vi "XYZArrayInverter.vi"(1 "input array":dbl[](array[numeric]), 2 "invert?":bool, 3 "Number":i32) -> (0 "modified array":dbl[](array[numeric]))   [LabVIEW 2015]
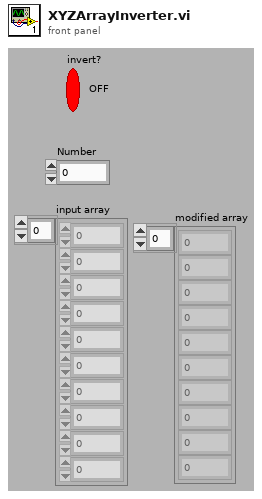
[diagram p1: front panel]
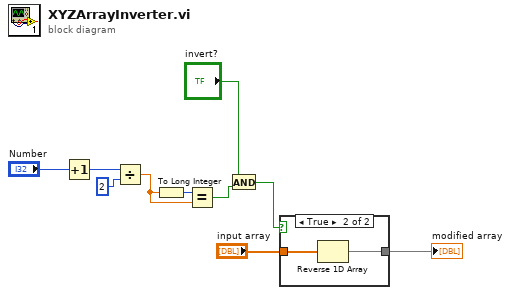
[diagram p0: block diagram]
diagram:
  n1 = Increment(x="Number") -> (x+1=w4:i32)
  n2 = Divide(x=w4, y=2) -> (x/y=w7:dbl)
  n3 = To Long Integer(number=w7) -> (32bit integer=w6:i32)
  n4 = Equal?(x=w6, y=w7) -> (x = y?=w3:bool)
  n5 = And(x="invert?", y=w3) -> (x .and. y?=w2:bool)
  n6 = case shown="True" w2 {
    tunnel: "input array" -> [w11 w13]
    tunnel: [w11 w12] -> w9
    frame False {
    }
    frame True {
      n7 = Reverse 1D Array(array=w13) -> (reversed array=w12:dbl[])
    }
  }
  "modified array" <- w9
